vi "ApplyLibraryIconToVIs.vi"(8 "error in (no error)":errorcluster, 11 "Library Refnum":refnum<vi>) -> (0 "error out":errorcluster, 3 "Library Refnum out":refnum<vi>)   [LabVIEW 2014, in "ClassIconTools.lvlib"]
uses:
  ClassIconTools.lvlib
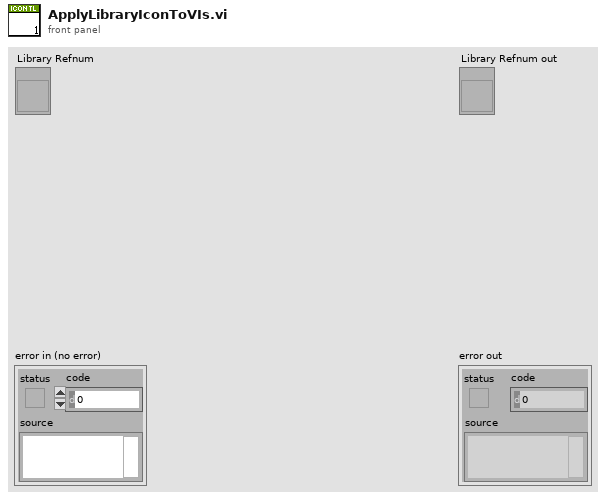
[diagram p1: front panel]
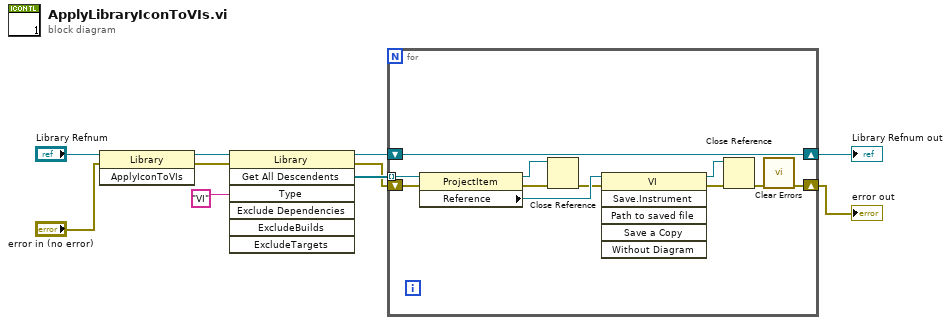
[diagram p0: block diagram]
diagram:
  n1 = invoke class="Library" method="ApplyIconToVIs"(reference="Library Refnum", error in="error in (no error)") -> (reference out=w8:refnum<vi>, error out=w5:errorcluster)  [unwired: 1 in, 1 out]
  n2 = invoke class="Library" method="Get All Descendents"(reference=w8, error in=w5, "Type"="VI") -> (reference out=w9:refnum<vi>, error out=w3:errorcluster, "All Descendents"=w10:refnum<vi>[])  [unwired: 4 in, 4 out]
  n3 = for {
    tunnel: w10 -> [w21] mode=indexing
    shift-right: [w17] -> w2
    shift-left: w9 -> [w17]
    shift-right: [w11] -> w1
    shift-left: w3 -> [w16]
    n4 = property class="ProjectItem"(reference=w21, error in=w16) -> (reference out=w18:refnum<vi>, error out=w15:errorcluster, "Reference"=w20:refnum<vi>)
    n5 = Close Reference(reference=w18, error in (no error)=w15) -> (error out=w14:errorcluster)
    n6 = invoke class="VI" method="Save.Instrument"(reference=w20, error in=w14) -> (reference out=w19:refnum<vi>, error out=w13:errorcluster)  [unwired: 4 in, 4 out]
    n7 = Close Reference(reference=w19, error in (no error)=w13) -> (error out=w12:errorcluster)
    n8 = call <vilib>:"Clear Errors.vi"("error in (no error)"=w12) -> ("error out"=w11:errorcluster)  [unwired: 5 in, 1 out]
  }
  "error out" <- w1
  "Library Refnum out" <- w2
